vi "Wait For Acquisition_LeCroy.vi"(8 "error in (no error)":errorcluster, 10 "Timeout (10000 ms)":u32=10000, 11 "VISA resource name":refnum<visa-resource-name>) -> (0 "error out":errorcluster, 2 "Complete":bool, 3 "VISA resource name out":refnum<visa-resource-name>)   [LabVIEW 2022 SP3]
doc: "This detect whether previous operation finished in specified time or no."
uses:
  <instrlib>/LeCroy Wave Series/LeCroy Wave Series.lvlib
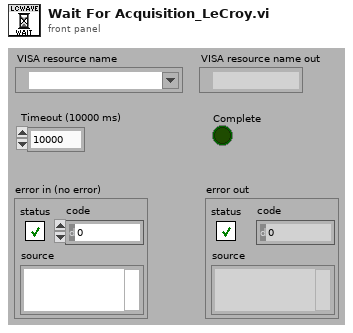
[diagram p1: front panel]
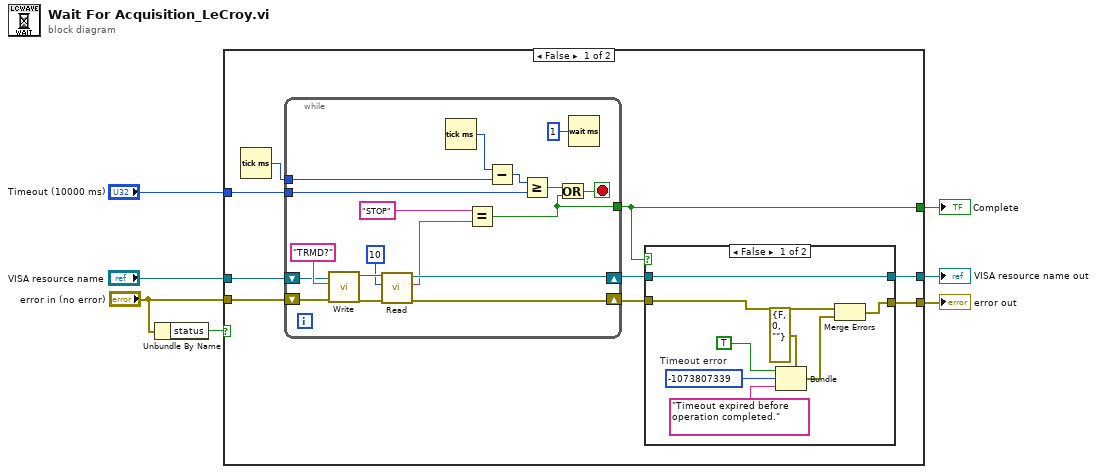
[diagram p0: block diagram]
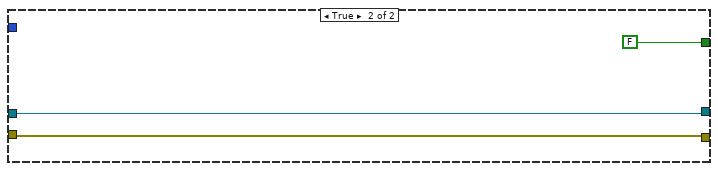
[diagram p3: hidden frame]
diagram:
  n1 = Unbundle By Name("error in (no error)") -> ("status"=w2:bool)
  n2 = case shown="False" w2 {
    tunnel: "VISA resource name" -> [w16 w47]
    tunnel: "Timeout (10000 ms)" -> [w14 _]
    tunnel: [w11 w47] -> w5
    tunnel: [w10 w46] -> w4
    tunnel: "error in (no error)" -> [w9 w46]
    tunnel: [w8 FALSE] -> w1
    frame False {
      n3 = Tick Count (ms)() -> (millisecond timer value=w15:u32)
      n4 = while {
        tunnel: w15 -> [w37]
        tunnel: w14 -> [w35]
        tunnel: [w27] -> w8
        shift-right: [w31] -> w13
        shift-left: w16 -> [w40]
        shift-right: [w30] -> w12
        shift-left: w9 -> [w39]
        stop <- w34 stop-if-true
        n5 = call <instrlib>:"Write.vi"("error in (no error)"=w39, "Write Buffer"="TRMD?" ("write buffer"), "VISA resource name"=w40) -> ("error out"=w43:errorcluster, "VISA resource name out"=w44:refnum<visa-resource-name>)  [unwired: 6 in, 1 out]
        n6 = call <instrlib>:"Read.vi"("error in (no error)"=w43, "Byte Count"=u32 10 ("byte count"), "VISA resource name"=w44) -> ("error out"=w30:errorcluster, "Read Buffer"=w28:string, "VISA resource name out"=w31:refnum<visa-resource-name>)  [unwired: 5 in, 1 out]
        n7 = Tick Count (ms)() -> (millisecond timer value=w38:u32)
        n8 = Equal?(x="STOP" ("write buffer"), y=w28) -> (x = y?=w27:bool)
        n9 = Subtract(x=w38, y=w37) -> (x-y=w36:u32)
        n10 = Greater Or Equal?(x=w36, y=w35) -> (x >= y?=w33:bool)
        n11 = Or(x=w33, y=w27) -> (x .or. y?=w34:bool)
        n12 = Wait (ms)(milliseconds to wait=u32 1) -> ()  [unwired: 1 out]
      }
      n13 = case shown="False" w8 {
        tunnel: w13 -> [w20 w26]
        tunnel: w12 -> [w18 w25]
        tunnel: [w20 w26] -> w11
        tunnel: [w19 w25] -> w10
        frame False {
          w23 = -1073807339  # Timeout error
          n14 = Bundle(cluster=errorcluster {"status"=FALSE, "code"=0, "source"=""} ("error out"), "status"=TRUE, "code"=w23, "source"="Timeout expired before operation completed." ("Source")) -> (w17:errorcluster)
          n15 = Merge Errors(w18, w17) -> (w19:errorcluster)
        }
        frame True {
        }
      }
    }
    frame True {
    }
  }
  "VISA resource name out" <- w5
  "error out" <- w4
  "Complete" <- w1
